vi "Terminal_Velocity_Viscous.vi"() -> ()   [LabVIEW 2022 SP3]
panel:
  out "Terminal Velocity (m/s)":dbl
  in  "Fluid Viscosity (Ns/m^2)":dbl
  in  "Particle Radius (m)":dbl
  in  "Fluid Density (kg/m^3)":dbl
  in  "Particle Density (kg/m^3)":dbl
  # "Terminal_Velocity_Viscous:\nA particle in free fall will continue to speed up\nuntil its acceleration turns to 0. This terminal \nvelocity for a particle in a viscous fluid is calculated below.\nEnter the values for density of the particle (rho), viscosity of \nthe fluid (eta), density of the fluid (rhof), and radius of the \nparticle (r) to see the particle's terminal velocity."
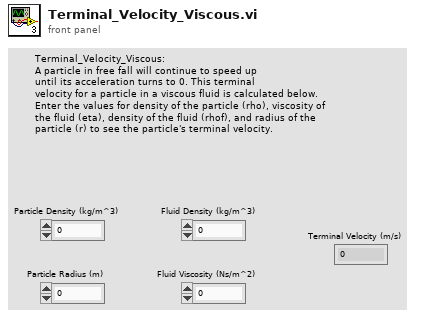
[diagram p1: front panel]
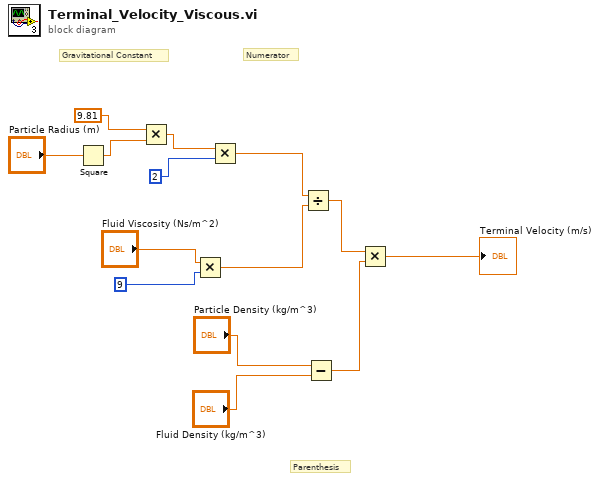
[diagram p0: block diagram]
diagram:
  # "Parenthesis"
  # "Numerator"
  # "Gravitational Constant"
  n1 = Square(x="Particle Radius (m)") -> (x^2=w10:dbl)
  n2 = Multiply(x=9.81, y=w10) -> (x*y=w9:dbl)
  n3 = Multiply(x="Fluid Viscosity (Ns/m^2)", y=9) -> (x*y=w4:dbl)
  n4 = Multiply(x=w9, y=2) -> (x*y=w5:dbl)
  n5 = Divide(x=w5, y=w4) -> (x/y=w3:dbl)
  n6 = Subtract(x="Particle Density (kg/m^3)", y="Fluid Density (kg/m^3)") -> (x-y=w2:dbl)
  n7 = Multiply(x=w3, y=w2) -> (x*y=→"Terminal Velocity (m/s)":dbl)
